vi "Generate Average Coverage String.vi"(8 "error in (no error)":errorcluster, 11 "Coverage Analyzer Result View in":refnum<class "Coverage Analyzer Result View.lvclass">) -> (0 "error out":errorcluster, 2 "Fraction of VIs Executed":string, 3 "Coverage Analyzer Result View out":refnum<class "Coverage Analyzer Result View.lvclass">)   [LabVIEW 2020, in "Coverage Analyzer Result View.lvclass"]
uses:
  Coverage Analyzer Result View.lvclass
  Coverage Analyzer Result View.lvclass/Coverage Analyzer Result View.ctl
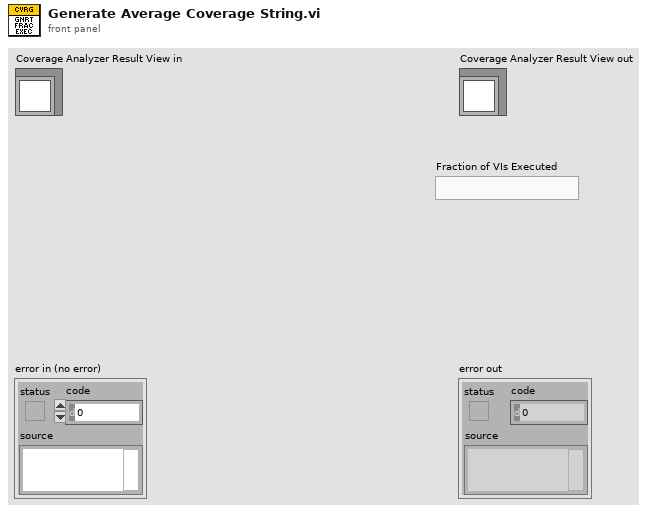
[diagram p1: front panel]
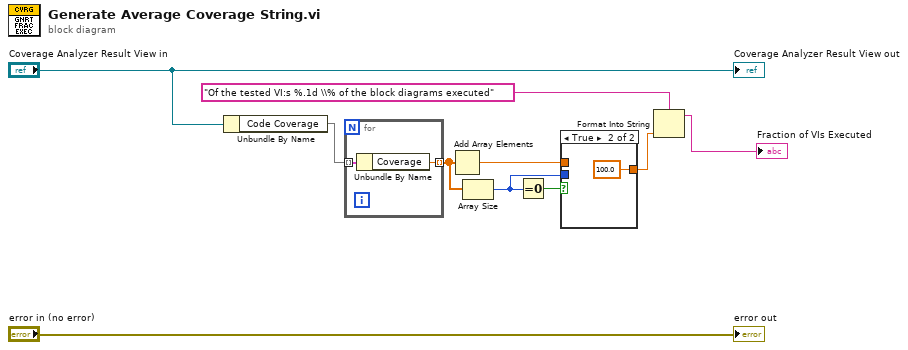
[diagram p0: block diagram]
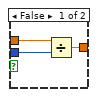
[diagram p2: hidden frame]
diagram:
  n1 = Unbundle By Name("Coverage Analyzer Result View in") -> ("Code Coverage"=w6:map{path, dbl})
  n2 = for {
    tunnel: w6 -> [w12] mode=indexing
    tunnel: [w11] -> w4 mode=indexing
    n3 = Unbundle By Name(w12) -> ("Coverage"=w11:dbl)
  }
  n4 = Add Array Elements(numeric array=w4) -> (sum=w5:dbl)
  n5 = Array Size(array=w4) -> (size(s)=w1:i32)
  n6 = Equal To 0?(x=w1) -> (x = 0?=w2:bool)
  n7 = case shown="True" w2 {
    tunnel: w5 -> [w15 _]
    tunnel: [w14 100.0] -> w3
    tunnel: w1 -> [w13 _]
    frame False {
      n8 = Divide(x=w15, y=w13) -> (x/y=w14:dbl)
    }
    frame True {
    }
  }
  n9 = Format Into String(format string="Of the tested VI:s %.1d \\% of the block diagrams executed", w3) -> (resulting string=→"Fraction of VIs Executed":string)  [unwired: 2 in, 1 out]
  "error out" <- "error in (no error)"
  "Coverage Analyzer Result View out" <- "Coverage Analyzer Result View in"
